vi "Channel_Writter.vi"() -> ()   [LabVIEW 2017]
uses:
  <extravilib>/ChannelInstances/Stream-dbl/Read With Abort.vi
  <extravilib>/ChannelInstances/Stream-dbl/Write With Abort.vi
  <extravilib>/ChannelInstances/Stream-dbl/EndpointRead.vi
  <extravilib>/ChannelInstances/Stream-dbl/Endpoint.vi
  <extravilib>/ChannelInstances/Stream-dbl/Instantiate.vi
  <extravilib>/ChannelInstances/Stream-dbl/)Channel.vi
  <resource>/ChannelSupport/_ChannelSupport/WaitIfNeeded.vi
  <extravilib>/ChannelInstances/Stream-dbl.lvlib
panel:
  in  "milliseconds to wait 2":u32
  out "Waveform Chart 2":dbl(graph)
  in  "Stop Button 2":bool
  in  "milliseconds to wait":u32
  out "Waveform Chart":dbl(graph)
  in  "Stop Button":bool
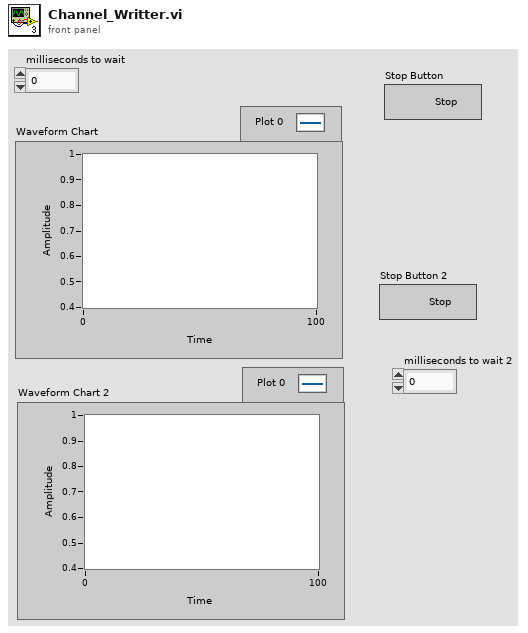
[diagram p1: front panel]
types:
  T1 = typedef "Stream-dbl.lvlib/)Channel.ctl" = refnum<queue>
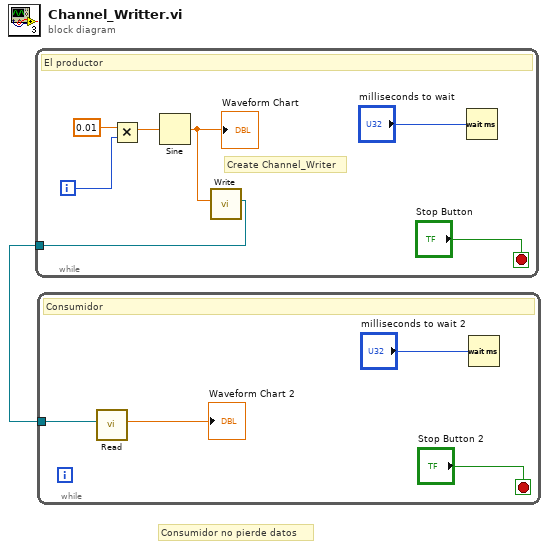
[diagram p0: block diagram]
diagram:
  # "Consumidor no pierde datos"
  n1 = while {
    tunnel: [w2] -> w1
    i -> [w6]
    stop <- "Stop Button" stop-if-true
    # "Create Channel_Writer"
    # "El productor"
    n2 = Multiply(x=0.01, y=w6) -> (x*y=w5:dbl)
    n3 = Sine(x=w5) -> (sin(x)=w3:dbl)
    "Waveform Chart" <- w3
    n4 = call <extravilib>:"Write.vi"("element"=w3) -> ("channel"=w2:T1)  [unwired: 8 in, 2 out]
    n5 = Wait (ms)(milliseconds to wait="milliseconds to wait") -> ()  [unwired: 1 out]
  }
  n6 = while {
    tunnel: w1 -> [w10]
    stop <- "Stop Button 2" stop-if-true
    # "Consumidor"
    n7 = call <extravilib>:"Read.vi"("channel"=w10) -> ("element"=→"Waveform Chart 2":dbl)  [unwired: 6 in, 4 out]
    n8 = Wait (ms)(milliseconds to wait="milliseconds to wait 2") -> ()  [unwired: 1 out]
  }
